vi "injector setpoint.vi"(8 "error in (no error)":errorcluster, 9 "set point":dbl, 10 "Pass setpoint?":u16, 11 "VISA Refnum in":refnum<visa-resource-name>) -> (0 "error out":errorcluster, 2 "MFC options":u16, 3 "VISA Refnum out":refnum<visa-resource-name>)   [LabVIEW 2016]
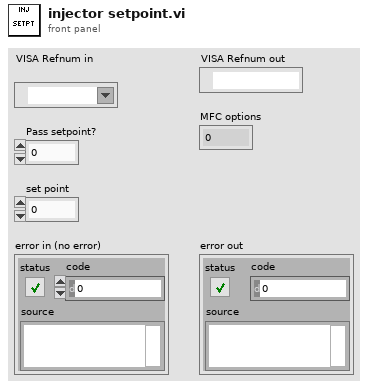
[diagram p1: front panel]
types:
  T1 = enum16{"Poll", "Set Stream", "Set Poll", "Define Set Point", "Gas Select", "Set P Gain", "Set D Gain", "Get P Gain", "Get D Gain", "Assign New Addess", ""}
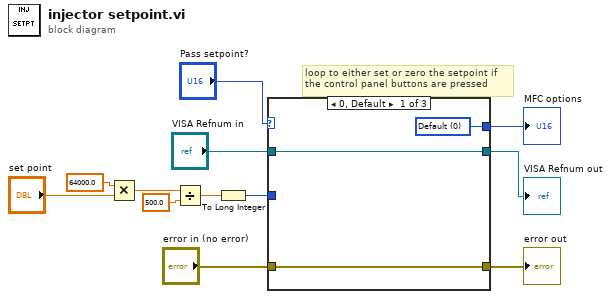
[diagram p0: block diagram]
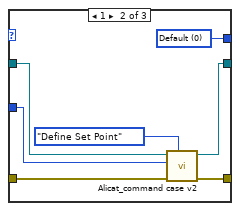
[diagram p2: hidden frame]
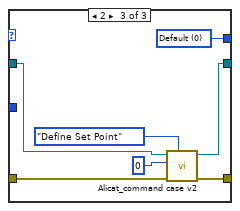
[diagram p3: hidden frame]
diagram:
  # "loop to either set or zero the setpoint if \nthe control panel buttons are pressed"
  n1 = Multiply(x=64000.0, y="set point") -> (x*y=w4:dbl)
  n2 = Divide(x=w4, y=500.0) -> (x/y=w6:dbl)
  n3 = To Long Integer(number=w6) -> (32bit integer=w7:i32)
  n4 = case shown="0, Default" "Pass setpoint?" {
    tunnel: [w14 w22 w29] -> w1
    tunnel: [w15 w21 w28] -> w2
    tunnel: w7 -> [_ w20 _]
    tunnel: "error in (no error)" -> [w15 w18 w25]
    tunnel: "VISA Refnum in" -> [w14 w17 w24]
    tunnel: [w13 w16 w23] -> w12
    frame 0, Default {
      w13 = u16 0 items=["Default", "Pass Set Point", "Reset"] ("MFC options")
    }
    frame 1 {
      w16 = u16 0 items=["Default", "Pass Set Point", "Reset"] ("MFC options")
      n5 = call "Alicat_command case v2.vi"("Case"=T1."Define Set Point", "error in (no error)"=w18, "Val 1"=w20, "VISA resource name"=w17) -> ("error out"=w21:errorcluster, "dup VISA resource name"=w22:refnum<visa-resource-name>)  [unwired: 4 in, 2 out]
    }
    frame 2 {
      w23 = u16 0 items=["Default", "Pass Set Point", "Reset"] ("MFC options")
      n6 = call "Alicat_command case v2.vi"("Case"=T1."Define Set Point", "error in (no error)"=w25, "Val 1"=0, "VISA resource name"=w24) -> ("error out"=w28:errorcluster, "dup VISA resource name"=w29:refnum<visa-resource-name>)  [unwired: 4 in, 2 out]
    }
  }
  "MFC options" <- w12
  "error out" <- w2
  "VISA Refnum out" <- w1
